vi "Main.vi"() -> ()   [LabVIEW 2019, in "HVC5.lvlib" / "HVC5.lvclass"]
uses:
  HVC5.lvclass
  typeDefs/Server State Data.ctl
  HVC5.lvclass/HVC5.ctl
panel:
  in  "Stop":bool
  in  "Enable Async Mode":bool
  in  "Server Address":string="0.0.0.0:50051"
  in  "Server Certificate File (.crt)":path
  in  "Server Key File (.key)":path
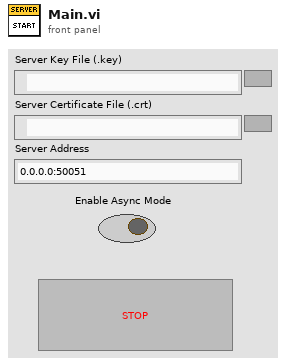
[diagram p1: front panel]
types:
  T1 = typedef "HVC5.lvlib/HVC5.lvclass/Server State Data.ctl" = cluster{"Data":string}
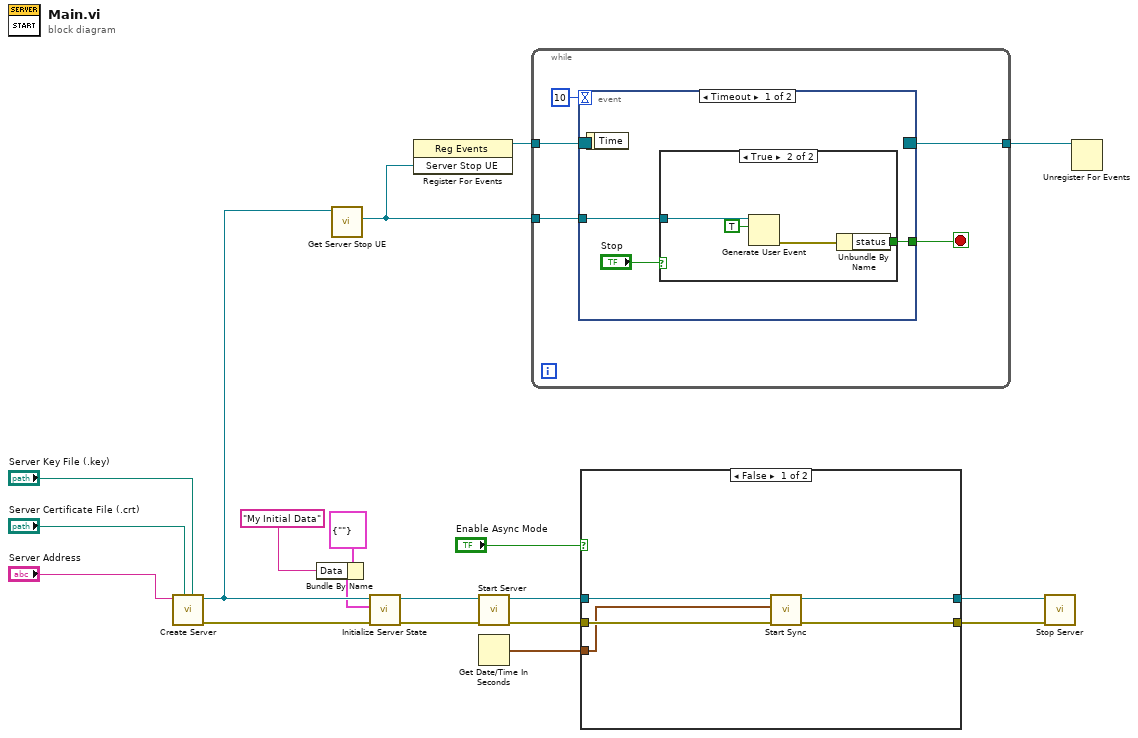
[diagram p0: block diagram]
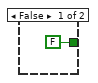
[diagram p2: hidden frame]
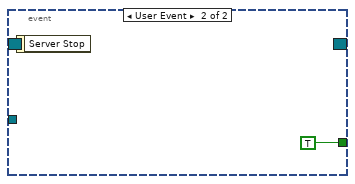
[diagram p3: hidden frame]
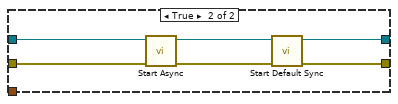
[diagram p4: hidden frame]
diagram:
  n1 = call "Create Server.vi"("Server Key File (.key)"="Server Key File (.key)", "Server Certificate File (.crt)"="Server Certificate File (.crt)", "Server Address"="Server Address") -> ("error out"=w8:errorcluster, "gRPC Server out"=w5:refnum<class "HVC5.lvclass">)  [unwired: 7 in]
  n2 = Bundle By Name(cluster=T1 {"Data"=""} ("Initial State"), "Data"="My Initial Data") -> (w3:T1)
  n3 = call "Get Server Stop UE.vi"("OOP Server in"=w5) -> ("Server Stop UE"=w9:refnum<user-event>)  [unwired: 9 in, 1 out]
  n4 = call "Initialize Server State.vi"("error in (no error)"=w8, "Initial State"=w3, "gRPC Server in"=w5) -> ("error out"=w7:errorcluster, "gRPC Server out"=w6:refnum<class "HVC5.lvclass">)  [unwired: 7 in]
  n5 = register-events(w9) -> (reference out=w11:refnum<event-registration>)  [unwired: 2 in, 1 out]
  n6 = call "Start Server.vi"("error in (no error)"=w7, "gRPC Server in"=w6) -> ("error out"=w19:errorcluster, "gRPC Server out"=w18:refnum<class "HVC5.lvclass">)  [unwired: 8 in]
  n7 = Get Date/Time In Seconds() -> (seconds since 1Jan1904=w1:timestamp)
  n8 = while {
    tunnel: w9 -> [w24]
    tunnel: w11 -> [w23]
    tunnel: [w21] -> w10
    stop <- w22 stop-if-true
    n9 = event shown="[0] Timeout" {
      selector: w23 -> [_ _]
      dyn-events: [_ _] -> w21
      timeout: 10 -> [_ _]
      tunnel: w24 -> [w26 _]
      tunnel: [w27 TRUE] -> w22
      event Timeout {
        n10 = event-data() -> ()  [unwired: 1 in, 1 out]
        n11 = case shown="True" "Stop" {
          tunnel: [FALSE ("status") w30] -> w27
          tunnel: w26 -> [_ w29]
          frame False {
          }
          frame True {
            n12 = Generate User Event(user event=w29, event data cluster=TRUE ("event data")) -> (error out=w31:errorcluster)  [unwired: 2 in, 1 out]
            n13 = Unbundle By Name(w31) -> ("status"=w30:bool)
          }
        }
      }
      event User Event {
        n14 = event-data() -> ()  [unwired: 1 in, 1 out]
      }
    }
  }
  n15 = case shown="False" "Enable Async Mode" {
    tunnel: w19 -> [w38 w44]
    tunnel: w18 -> [w37 w43]
    tunnel: [w36 w40] -> w17
    tunnel: [w35 w39] -> w16
    tunnel: w1 -> [w34 _]
    frame False {
      n16 = call "Start Sync.vi"("error in (no error)"=w38, "current time"=w34, "gRPC Server in"=w37) -> ("error out"=w36:errorcluster, "gRPC Server out"=w35:refnum<class "HVC5.lvclass">)  [unwired: 7 in]
    }
    frame True {
      n17 = call "Start Async.vi"("error in (no error)"=w44, "gRPC Server in"=w43) -> ("error out"=w41:errorcluster, "gRPC Server out"=w42:refnum<class "HVC5.lvclass">)  [unwired: 8 in]
      n18 = call "Start Default Sync.vi"("error in (no error)"=w41, "gRPC Server in"=w42) -> ("error out"=w40:errorcluster, "gRPC Server out"=w39:refnum<class "HVC5.lvclass">)  [unwired: 8 in]
    }
  }
  n19 = call "Stop Server.vi"("error in (no error)"=w17, "gRPC Server in"=w16) -> ()  [unwired: 9 in, 1 out]
  n20 = Unregister For Events(event registration refnum=w10) -> ()  [unwired: 1 in, 1 out]
